vi "Find Classes Out of Date.vi"(8 "error in (no error)":errorcluster, 11 "Test Finder In":refnum<class "Test Finder.lvclass">) -> (0 "error out":errorcluster, 2 "Outdated Test Class paths":path[](array[path]), 3 "Test Finder Out":refnum<class "Test Finder.lvclass">)   [LabVIEW 2020, in "Test Finder.lvclass"]
uses:
  Test Finder.lvclass
  Test Finder.lvclass/Test Finder.ctl
  <vilib>/security/Message Digest/API/Instances/File/SHA-256 File Checksum.vi
  <vilib>/security/Message Digest/API/NI_Message Digest API.lvlib
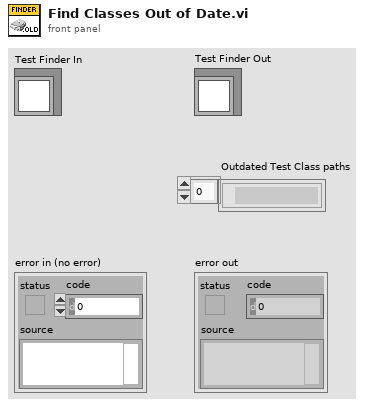
[diagram p1: front panel]
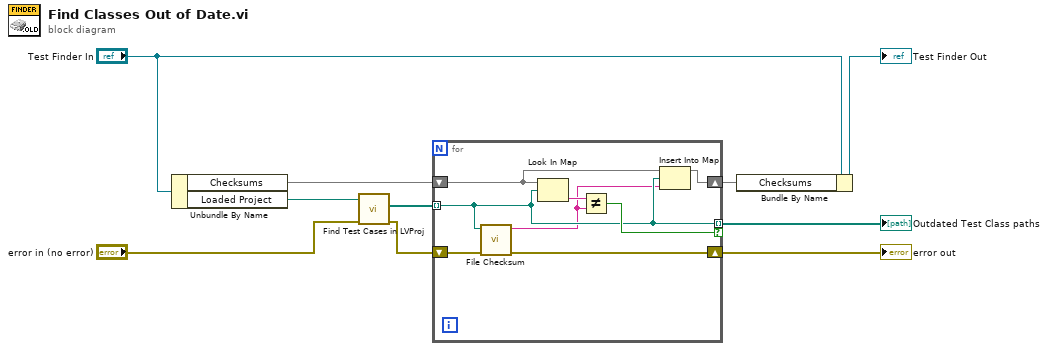
[diagram p0: block diagram]
diagram:
  n1 = Unbundle By Name("Test Finder In") -> ("Checksums"=w4:map{path, string}, "Loaded Project"=w9:path)
  n2 = call "Find Test Cases in LVProj.vi"("error in (no error)"="error in (no error)", "Project Path"=w9) -> ("error out"=w6:errorcluster, "Test Class paths"=w7:path[])  [unwired: 8 in]
  n3 = for {
    tunnel: w7 -> [w12] mode=indexing
    shift-right: [w17] -> w5
    shift-left: w6 -> [w18]
    tunnel: [w12] -> w3 mode=indexing if=w15
    shift-right: [w13] -> w1
    shift-left: w4 -> [w14]
    n4 = call-poly <vilib>:"File Checksum.vi"("error in"=w18, "path"=w12) -> ("error out"=w17:errorcluster, "digest"=w11:string)  [unwired: 8 in]
    n5 = Look In Map(map=w14, key=w12) -> (value=w16:string)  [unwired: 1 in, 1 out]
    n6 = Not Equal?(x=w16, y=w11) -> (x != y?=w15:bool)
    n7 = Insert Into Map(map in=w14, key=w12, value=w11) -> (map out=w13:map{path, string})  [unwired: 2 out]
  }
  "error out" <- w5
  "Outdated Test Class paths" <- w3
  n8 = Bundle By Name(cluster="Test Finder In", "Checksums"=w1) -> (→"Test Finder Out":refnum<class "Test Finder.lvclass">)
